vi "SetString_Message.vi"(6 "LastCalLocation":string="Oncore", 7 "PcbRevision":string="8", 8 "PcbAssemblyNum":string="EAP0226L50", 9 "ManufactLocation":string="Oncore", 10 "ManufactDate":string="02-06-2012", 11 "SerialNumb":string="test3") -> (5 "LastCalDate":string=" 5- 6-2012")   [LabVIEW 2013]
panel:
  in  "State":enum16{"Exit", "blankcheck", "empty"}(ring)
  in  "OK":bool
  # "VERIFY UUT INFORMATION"
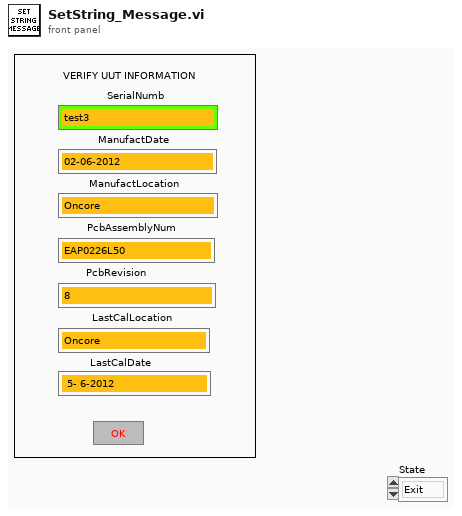
[diagram p1: front panel]
types:
  T1 = typedef "LVDateTimeRec.ctl" = cluster{"fractional second":dbl, "second":i32, "minute":i32, "hour":i32, "day of month":i32, "month":i32, "year":i32, "day of week":i32, "day of year":i32, "DST":i32}
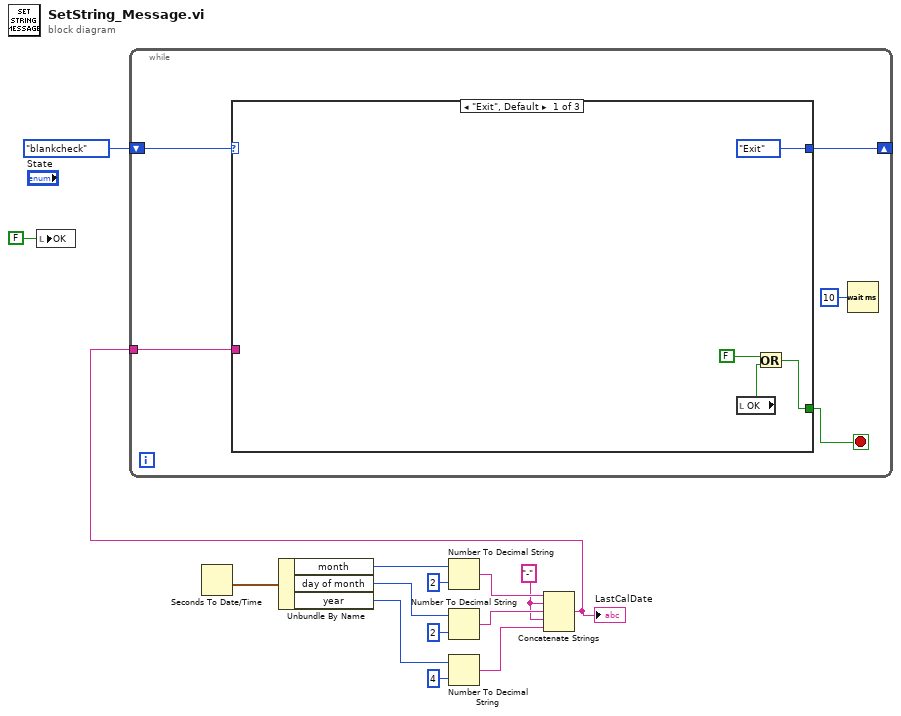
[diagram p0: block diagram]
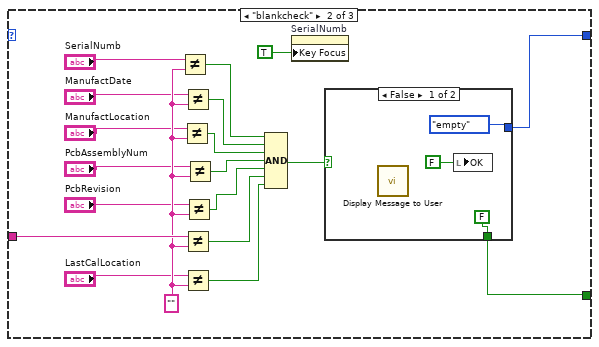
[diagram p2: hidden frame]
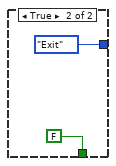
[diagram p3: hidden frame]
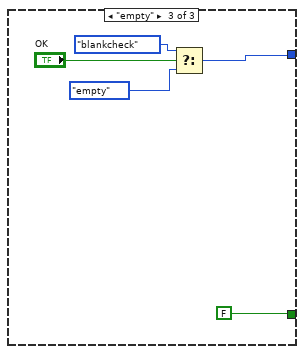
[diagram p4: hidden frame]
diagram:
  w4 = "-"
  n1 = local write "OK"(FALSE ("OK")) -> ()
  n2 = Seconds To Date/Time() -> (date time rec=w14:T1)  [unwired: 2 in]
  n3 = Unbundle By Name(w14) -> ("month"=w13:i32, "day of month"=w10:i32, "year"=w8:i32)
  n4 = Number To Decimal String(number=w13, width (-)=i16 2) -> (decimal integer string=w7:string)
  n5 = Number To Decimal String(number=w10, width (-)=i16 2) -> (decimal integer string=w6:string)
  n6 = Number To Decimal String(number=w8, width (-)=i16 4) -> (decimal integer string=w5:string)
  n7 = Concatenate Strings(w7, w4, w6, w4, w5) -> (w3:string)
  "LastCalDate" <- w3
  n8 = while {
    tunnel: w3 -> [w19]
    shift-right: [w16] -> _
    shift-left: enum16{"Exit", "blankcheck", "empty"}."blankcheck" ("State") -> [w17]
    stop <- w15 stop-if-true
    n9 = case shown="\"Exit\", Default" w17 {
      tunnel: w19 -> [_ w42 _]
      tunnel: [enum16{"Exit", "blankcheck", "empty"}."Exit" ("State") w26 w49] -> w16
      tunnel: [w20 w24 FALSE] -> w15
      frame "Exit", Default {
        n10 = local read "OK"() -> (w22:bool)
        n11 = Or(x=FALSE, y=w22) -> (x .or. y?=w20:bool)
      }
      frame "blankcheck" {
        w41 = ""
        n12 = Not Equal?(x="SerialNumb", y=w41) -> (x != y?=w40:bool)
        n13 = Not Equal?(x="ManufactLocation", y=w41) -> (x != y?=w38:bool)
        n14 = Not Equal?(x="ManufactDate", y=w41) -> (x != y?=w39:bool)
        n15 = Not Equal?(x=w42, y=w41) -> (x != y?=w35:bool)
        n16 = Not Equal?(x="LastCalLocation", y=w41) -> (x != y?=w34:bool)
        n17 = Not Equal?(x="PcbRevision", y=w41) -> (x != y?=w36:bool)
        n18 = Not Equal?(x="PcbAssemblyNum", y=w41) -> (x != y?=w37:bool)
        n19 = Compound Arithmetic op=AND(w40, w39, w38, w37, w36, w35, w34) -> (w27:bool)
        n20 = property on="SerialNumb" class="Str"("Key Focus"=TRUE) -> ()  [unwired: 2 in, 2 out]
        n21 = case shown="False" w27 {
          tunnel: [FALSE FALSE] -> w24
          tunnel: [enum16{"Exit", "blankcheck", "empty"}."empty" ("State") enum16{"Exit", "blankcheck", "empty"}."Exit" ("State")] -> w26
          frame False {
            n22 = call "Display Message to User"() -> ()  [unwired: 10 in, 2 out]
            n23 = local write "OK"(FALSE ("OK")) -> ()
          }
          frame True {
          }
        }
      }
      frame "empty" {
        n24 = Select(t=enum16{"Exit", "blankcheck", "empty"}."blankcheck" ("State"), s="OK", f=enum16{"Exit", "blankcheck", "empty"}."empty" ("State")) -> (s? t:f=w49:enum16{"Exit", "blankcheck", "empty"})
      }
    }
    n25 = Wait (ms)(milliseconds to wait=u32 10) -> ()  [unwired: 1 out]
  }
